vi "VARGLOB.vi"() -> ()   [LabVIEW 2021]
uses:
  VGLOBAL.vi
panel:
  in  "stop":bool
  out "Boolean":bool
  out "Waveform Chart":dbl(graph)
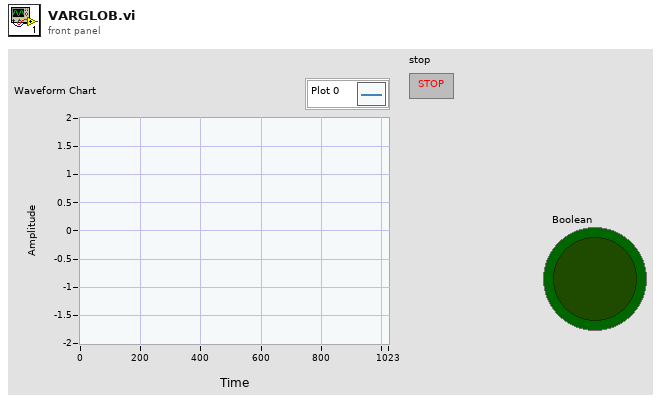
[diagram p1: front panel]
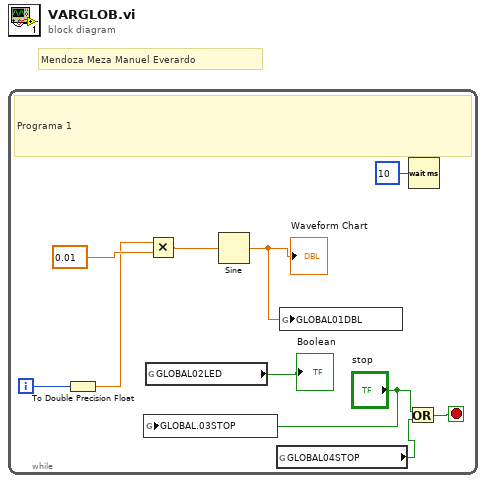
[diagram p0: block diagram]
diagram:
  # "Mendoza Meza Manuel Everardo"
  n1 = while {
    i -> [w8]
    stop <- w2 stop-if-true
    # "Programa 1"
    n2 = To Double Precision Float(number=w8) -> (double precision float=w7:dbl)
    n3 = global write "VGLOBAL.vi" "GLOBAL.03STOP"("stop") -> ()
    n4 = global read "VGLOBAL.vi" "GLOBAL02LED"() -> (→"Boolean":bool)
    n5 = Multiply(x=w7, y=0.01) -> (x*y=w6:dbl)
    n6 = Sine(x=w6) -> (sin(x)=w5:dbl)
    "Waveform Chart" <- w5
    n7 = global read "VGLOBAL.vi" "GLOBAL04STOP"() -> (w3:bool)
    n8 = global write "VGLOBAL.vi" "GLOBAL01DBL"(w5) -> ()
    n9 = Or(x="stop", y=w3) -> (x .or. y?=w2:bool)
    n10 = Wait (ms)(milliseconds to wait=u32 10) -> ()  [unwired: 1 out]
  }
